vi "Transmit.vi"(7 "packet? (f)":bool, 8 "error in (no error)":errorcluster, 10 "data":string, 11 "Socket.TCP in":refnum<class "Socket.TCP.lvclass">) -> (0 "error out":errorcluster, 2 "bytes written":i32, 3 "Socket.TCP out":refnum<class "Socket.TCP.lvclass">)   [LabVIEW 2014, in "Socket.lvlib" / "Socket.TCP.lvclass"]
doc: "socket.tcp.Transmit (data, packet?) Transmits the data, returns the number of bytes transmitted\n\nstring data\n\nbool packet? \nDefaults to false. If true, will prepend the data with two bytes indicating the size of the ata to follow (not including the size bytes)"
uses:
  Socket.TCP.lvclass
  Socket.TCP.lvclass/Socket.TCP.ctl
  Socket.Base/Socket.Base.lvclass/Socket.Base.ctl
  Accessors/Read tcp _refnum.vi
  Socket.Base/Accessors/Read timeout.vi
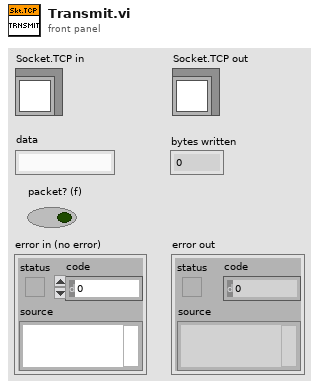
[diagram p1: front panel]
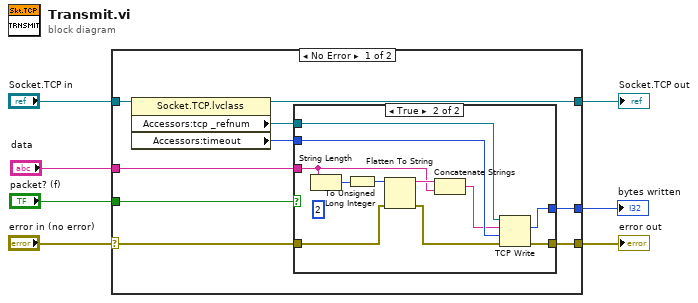
[diagram p0: block diagram]
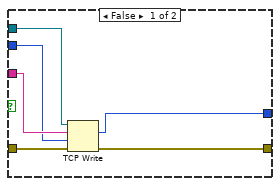
[diagram p2: hidden frame]
diagram:
  n1 = case shown="No Error" "error in (no error)" {
    selector: "error in (no error)" -> [w14 w35]
    tunnel: [w10 w35] -> w6
    tunnel: [w8 w34] -> w4
    tunnel: "Socket.TCP in" -> [w15 w34]
    tunnel: "packet? (f)" -> [w16 _]
    tunnel: "data" -> [w13 _]
    tunnel: [w9 _] -> w1
    frame No Error {
      n2 = property class="Socket.TCP.lvclass"(reference=w15) -> (reference out=w8:refnum<class "Socket.TCP.lvclass">, "Accessors:tcp _refnum"=w12:refnum<k5>, "Accessors:timeout"=w11:i32)  [unwired: 1 in, 1 out]
      n3 = case shown="True" w16 {
        tunnel: w14 -> [w22 w28]
        tunnel: w13 -> [w21 w23]
        tunnel: w12 -> [w20 w27]
        tunnel: w11 -> [w19 w32]
        tunnel: [w17 w31] -> w10
        tunnel: [w18 w30] -> w9
        frame False {
          n4 = TCP Write(connection ID=w20, data in=w21, error in (no error)=w22, 9:w19) -> (bytes written=w18:i32, error out=w17:errorcluster)  [unwired: 1 out]
        }
        frame True {
          (unwired) i16 2 ("width (-)")
          n5 = String Length(string=w23) -> (length=w33:i32)
          n6 = To Unsigned Long Integer(number=w33) -> (unsigned 32bit integer=w29:u32)
          n7 = Flatten To String(anything=w29, error in (no error)=w28) -> (data string=w24:string, error out=w26:errorcluster)  [unwired: 2 in, 1 out]
          n8 = Concatenate Strings(w24, w23) -> (w25:string)
          n9 = TCP Write(connection ID=w27, data in=w25, error in (no error)=w26, 9:w32) -> (bytes written=w30:i32, error out=w31:errorcluster)  [unwired: 1 out]
        }
      }
    }
    frame Error {
    }
  }
  "error out" <- w6
  "Socket.TCP out" <- w4
  "bytes written" <- w1
